vi "calculate binning.vi"(8 "error in (no error)":errorcluster, 10 "Value":dbl, 11 "Refnum in":T1) -> (0 "error out":errorcluster, 3 "Numeric":dbl)   [LabVIEW 2011]
uses:
  <vilib>/vision/Image Controls.llb/IMAQ Image.ctl
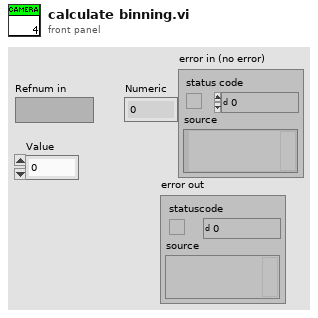
[diagram p1: front panel]
types:
  T1 = typedef "IMAQ Image.ctl" = refnum<image>
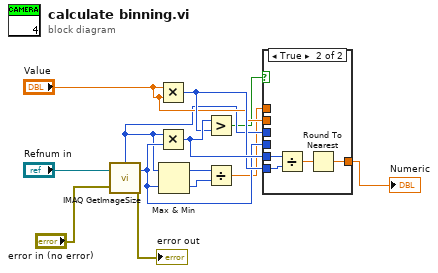
[diagram p0: block diagram]
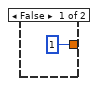
[diagram p2: hidden frame]
diagram:
  n1 = call "IMAQ GetImageSize"("Image"="Refnum in", "error in (no error)"="error in (no error)") -> ("Y Resolution"=w9:i32, "X Resolution"=w8:i32, "error out"=→"error out":errorcluster)  [unwired: 2 in]
  n2 = Multiply(x="Value", y="Value") -> (x*y=w11:u64)
  n3 = Multiply(x=w8, y=w9) -> (x*y=w12:u64)
  n4 = Max & Min(x=w8, y=w9) -> (max(x,y)=w5:i32, min(x,y)=w3:i32)
  n5 = Greater?(x=w12, y=w11) -> (0:w6:bool)
  n6 = Divide(x=w5, y=w3) -> (x/y=w4:dbl)
  n7 = case shown="True" w6 {
    tunnel: w4 -> [_ _]
    tunnel: "Value" -> [_ _]
    tunnel: w8 -> [_ _]
    tunnel: w9 -> [_ _]
    tunnel: [1 w17] -> w7
    tunnel: w11 -> [_ w16]
    tunnel: w12 -> [_ w15]
    frame False {
    }
    frame True {
      n8 = Divide(x=w15, y=w16) -> (x/y=w18:dbl)
      n9 = Round To Nearest(number=w18) -> (nearest integer value=w17:dbl)
    }
  }
  "Numeric" <- w7
